vi "Write Subscription Policy Settings.vi"(8 "Value Changes Only? (F)":bool, 9 "Boot Subscriber On Transport Failure? (T)":bool=TRUE, 10 "Ignore Past Updates? (F)":bool, 11 "SubscriptionPolicy in":refnum<class "SubscriptionPolicy.lvclass">) -> (3 "SubscriptionPolicy out":refnum<class "SubscriptionPolicy.lvclass">)   [LabVIEW 2015, in "IMediator.lvlib" / "SubscriptionPolicy.lvclass"]
uses:
  SubscriptionPolicy.lvclass
  SubscriptionPolicy.lvclass/SubscriptionPolicy.ctl
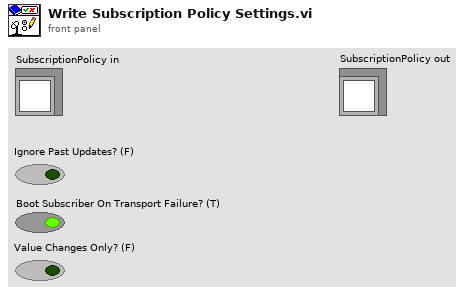
[diagram p1: front panel]
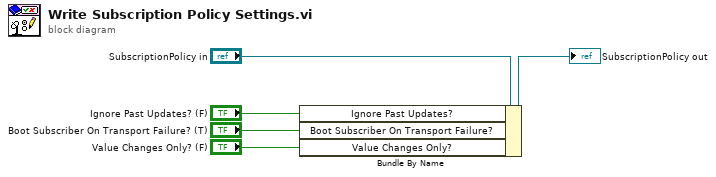
[diagram p0: block diagram]
diagram:
  n1 = Bundle By Name(cluster="SubscriptionPolicy in", "Ignore Past Updates?"="Ignore Past Updates? (F)", "Boot Subscriber On Transport Failure?"="Boot Subscriber On Transport Failure? (T)", "Value Changes Only?"="Value Changes Only? (F)") -> (→"SubscriptionPolicy out":refnum<class "SubscriptionPolicy.lvclass">)
